vi "Core Action.vi"(8 "error in (no error)":errorcluster, 10 "SECS-II Class":refnum<class "SECS-II Class.lvclass">, 11 "13-EnableDisable Alarm in":refnum<class "13-EnableDisable Alarm.lvclass">) -> (0 "error out":errorcluster, 2 "SECS-II Class Out":refnum<class "SECS-II Class.lvclass">, 3 "13-EnableDisable Alarm out":refnum<class "13-EnableDisable Alarm.lvclass">)   [LabVIEW 2020, in "SECS Scenarios.lvlib" / "13-EnableDisable Alarm.lvclass"]
uses:
  13-EnableDisable Alarm.lvclass
  D:/Dropbox/SECS/SECS_GEM v1.1.0/Com/SECS Scenarios/Scenarios Class/Scenarios Class.lvclass
  SECS Communication/SECS-II Class/SECS-II Class.lvclass
  SECS Communication/S5 Message Class/S5 Message Class.lvclass
  D:/Dropbox/SECS/SECS_GEM v1.1.0/Com/SECS Communication/SECS-II Class/SECS-II Class.lvclass
  Scenarios Class/Reply State.ctl
  Scenarios Class/Scenarios Class.lvclass/Scenarios Class.ctl
  Scenarios Class/Write Reply State.vi
  Scenarios Class/Read HSMS Class.vi
  SECS Communication/SECS Data Class/Get ALID Data.vi
  SECS Communication/SECS Data Class/Put ALID Data.vi
  SECS Communication/HSMS Class/HSMS Class.lvclass
  Scenarios Class/Scenarios Class.lvclass
  SECS Communication/SECS Data Class/SECS Data Class.lvclass
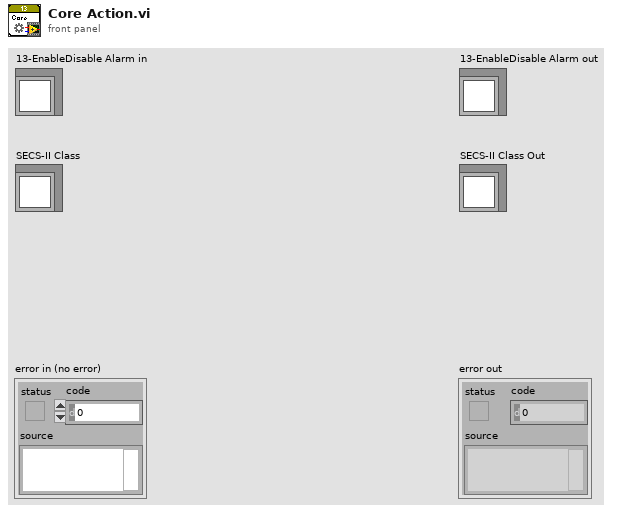
[diagram p1: front panel]
types:
  T1 = typedef "SECS Communication.lvlib/S5 Message Class.lvclass/S5F3.ctl" = cluster{"ALED":bool, "ALID":u32}
  T2 = typedef "SECS Scenarios.lvlib/Scenarios Class.lvclass/Reply State.ctl" = enum16{"OK", "Illegal Data", "Unknown Stream", "Unknown Function", "Off-Line", "T3 Timeout", "Inner-Timeout"}
  T3 = typedef "SECS Communication.lvlib/SECS Data Class.lvclass/ALID Data.ctl" = cluster{"Enable":bool, "ALID":u32, "Name":string, "Description":string, "Source":string, "Status":enum16{"Null", "Normal", "Abnormal", "Warning"}}
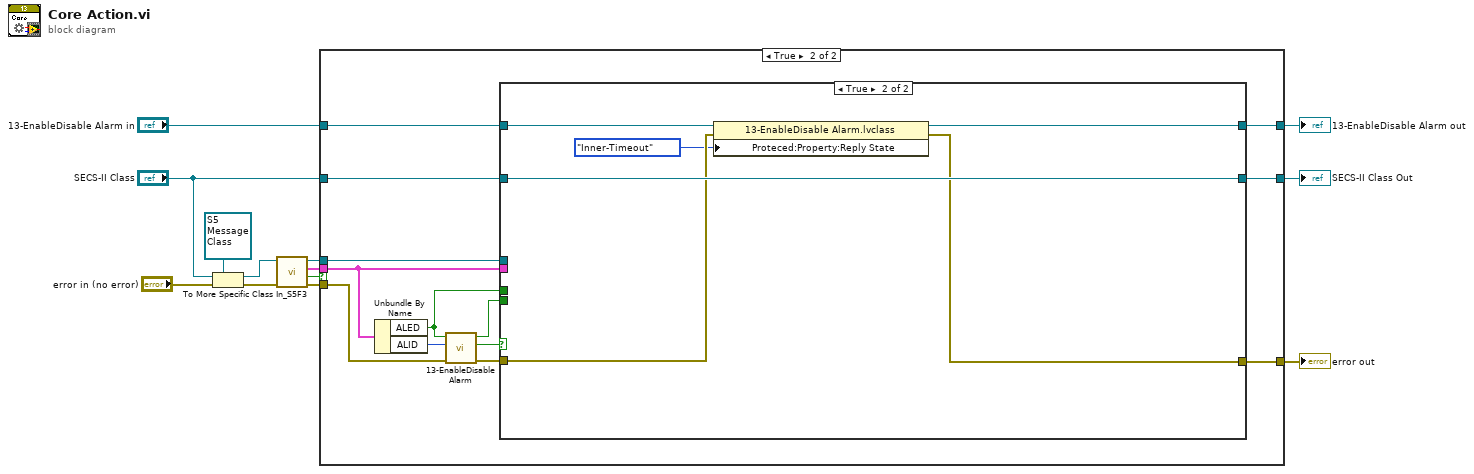
[diagram p0: block diagram]
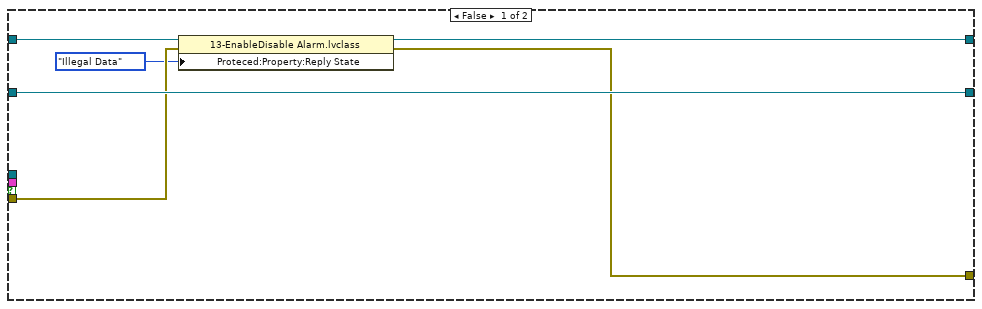
[diagram p2: hidden frame]
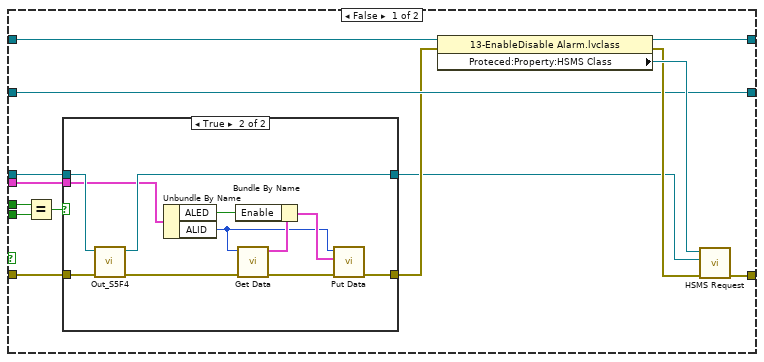
[diagram p3: hidden frame]
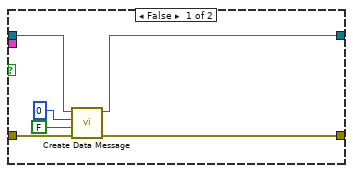
[diagram p4: hidden frame]
diagram:
  n1 = To More Specific Class(target class=refnum<class "S5 Message Class.lvclass"> refnum ("SECS Communication.lvlib:S5 Message Class.lvclass"), reference="SECS-II Class", error in="error in (no error)") -> (specific class reference=w10:refnum<class "S5 Message Class.lvclass">, error out=w11:errorcluster)
  n2 = call "In_S5F3.vi"("error in (no error)"=w11, "S5 Message Class in"=w10) -> ("error out"=w4:errorcluster, "OK?"=w1:bool, "S5F3"=w9:T1, "S5 Message Class out"=w8:refnum<class "S5 Message Class.lvclass">)  [unwired: 6 in]
  n3 = case shown="True" w1 {
    tunnel: "13-EnableDisable Alarm in" -> [w18 w32]
    tunnel: w9 -> [_ w20]
    tunnel: w8 -> [_ w31]
    tunnel: [w15 w30] -> w7
    tunnel: [w14 w29] -> w6
    tunnel: w4 -> [w17 w24]
    tunnel: "SECS-II Class" -> [w19 w23]
    tunnel: [w19 w22] -> w2
    frame False {
      n4 = property class="13-EnableDisable Alarm.lvclass"(reference=w18, error in=w17, "Proteced:Property:Reply State"=Reply_State."Illegal Data" ("Reply State")) -> (reference out=w15:refnum<class "13-EnableDisable Alarm.lvclass">, error out=w14:errorcluster)
    }
    frame True {
      n5 = Unbundle By Name(w20) -> ("ALED"=w21:bool, "ALID"=w28:u32)
      n6 = call "13-EnableDisable Alarm.vi"("error in (no error)"=w24, "ALID"=w28, "ALED"=w21) -> ("error out"=w27:errorcluster, "Timeout?"=w26:bool, "Enable"=w25:bool)  [unwired: 6 in]
      n7 = case shown="True" w26 {
        tunnel: w32 -> [w46 w68]
        tunnel: w31 -> [w39 _]
        tunnel: [w43 w66] -> w29
        tunnel: [w42 w67] -> w30
        tunnel: w27 -> [w40 w65]
        tunnel: w25 -> [w34 _]
        tunnel: w23 -> [w41 w69]
        tunnel: [w41 w69] -> w22
        tunnel: w21 -> [w37 _]
        tunnel: w20 -> [w33 _]
        frame False {
          n8 = Equal?(x=w37, y=w34) -> (x = y?=w36:bool)
          n9 = case shown="True" w36 {
            tunnel: w40 -> [w52 w63]
            tunnel: w39 -> [w51 w62]
            tunnel: [w50 w53] -> w38
            tunnel: [w47 w61] -> w35
            tunnel: w33 -> [_ w60]
            frame False {
              n10 = call "Create Data Message.vi"("error in (no error)"=w52, "W-Bit"=FALSE, "Function"=u8 0, "SECS-II Class in"=w51) -> ("error out"=w50:errorcluster, "SECS-II Class out"=w47:refnum<class "S5 Message Class.lvclass">)  [unwired: 6 in]
            }
            frame True {
              n11 = call "Out_S5F4.vi"("error in (no error)"=w63, "S5 Message Class in"=w62) -> ("error out"=w59:errorcluster, "S5 Message Class out"=w61:refnum<class "S5 Message Class.lvclass">)  [unwired: 8 in]
              n12 = Unbundle By Name(w60) -> ("ALED"=w57:bool, "ALID"=w54:u32)
              n13 = call-poly "Get Data.vi"("error in"=w59, "ALID"=w54) -> ("error out"=w56:errorcluster, "ALID Data"=w58:T3)  [unwired: 7 in, 1 out]
              n14 = Bundle By Name(cluster=w58, "Enable"=w57) -> (w55:T3)
              n15 = call-poly "Put Data.vi"("error in"=w56, "ALID Data"=w55, "ALID"=w54) -> ("error out"=w53:errorcluster)  [unwired: 7 in, 1 out]
            }
          }
          n16 = property class="13-EnableDisable Alarm.lvclass"(reference=w46, error in=w38) -> (reference out=w42:refnum<class "13-EnableDisable Alarm.lvclass">, error out=w44:errorcluster, "Proteced:Property:HSMS Class"=w45:refnum<class "HSMS Class.lvclass">)
          n17 = call "HSMS Request.vi"("error in (no error)"=w44, "SECS-II Class In"=w35, "HSMS Class in"=w45) -> ("error out"=w43:errorcluster)  [unwired: 7 in, 1 out]
        }
        frame True {
          n18 = property class="13-EnableDisable Alarm.lvclass"(reference=w68, error in=w65, "Proteced:Property:Reply State"=Reply_State."Inner-Timeout" ("Reply State")) -> (reference out=w67:refnum<class "13-EnableDisable Alarm.lvclass">, error out=w66:errorcluster)
        }
      }
    }
  }
  "error out" <- w6
  "13-EnableDisable Alarm out" <- w7
  "SECS-II Class Out" <- w2
